vi "Transform2d_GetRotation.vi"(11 "inTRANSFORM":T2={"TRANSLATION"={"X"=0.0, "Y"=0.0}, "ROTATION"={"VALUE"=0.0, "COS"=1.0, "SIN"=0.0}, "xF"=FALSE} {"ROTATION"."SIN" format="%13.4f"; "ROTATION"."COS" format="%13.4f"; "ROTATION"."VALUE" format="%13.4f"; "TRANSLATION"."Y" format="%14.3f"; "TRANSLATION"."X" format="%14.3f"}) -> (3 "ROTATION":T1={"VALUE"=0.0, "COS"=1.0, "SIN"=0.0} {"SIN" format="%13.4f"; "COS" format="%13.4f"; "VALUE" format="%13.4f"})   [LabVIEW 2019, in "Trajectory_Library.lvlib"]
doc: "Returns the rotational component of the transformation.\n\nParameters:\n - IN TRANSFORM - The TRANSFORM data structure\n\nReturns:\n - ROTATION - The rotational component of the transform."
uses:
  Trajectory_Library.lvlib
  TRANSFORM2D.ctl
  TRANSLATION2D.ctl
  ROTATION2D.ctl
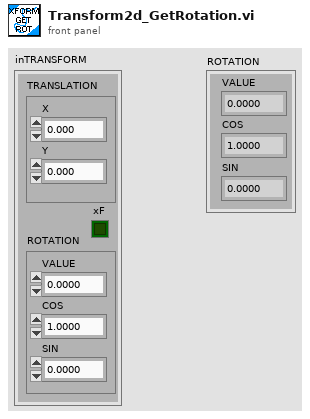
[diagram p1: front panel]
types:
  T1 = typedef "Trajectory_Library.lvlib/ROTATION2D.ctl" = cluster{"VALUE":dbl, "COS":dbl, "SIN":dbl}
  T2 = typedef "Trajectory_Library.lvlib/TRANSFORM2D.ctl" = cluster{"TRANSLATION":T3, "ROTATION":T1, "xF":bool}
  T3 = typedef "Trajectory_Library.lvlib/TRANSLATION2D.ctl" = cluster{"X":dbl, "Y":dbl}
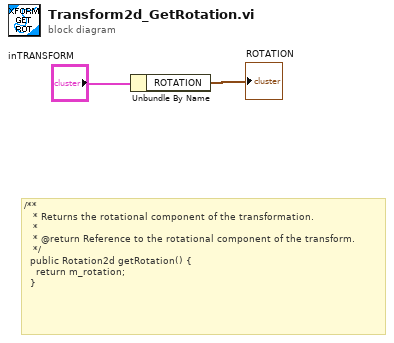
[diagram p0: block diagram]
diagram:
  # "/**\n   * Returns the rotational component of the transformation.\n   *\n   * @return Reference to the rotational component of the transform.\n   */\n  public Rotation2d getRotation() {\n    return m_rotation;\n  }"
  n1 = Unbundle By Name("inTRANSFORM") -> ("ROTATION"=→"ROTATION":T1)
